vi "Read CategoriesChanged Event.vi"(8 "error in (no error)":errorcluster, 11 "VIStore in":refnum<class "VIStore.lvclass">) -> (0 "error out":errorcluster, 2 "CatList Changed Event":refnum<user-event>, 3 "VIStore out":refnum<class "VIStore.lvclass">)   [LabVIEW 2015, in "VI App Store.lvlib" / "VIStore.lvclass"]
uses:
  VIStore.lvclass
  VIStore.lvclass/VIStore.ctl
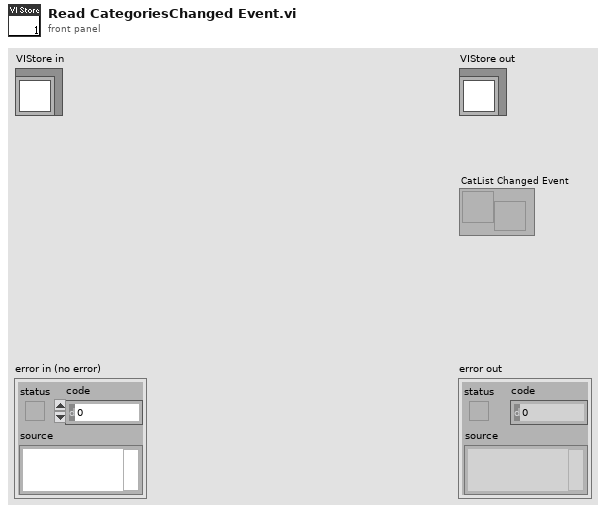
[diagram p1: front panel]
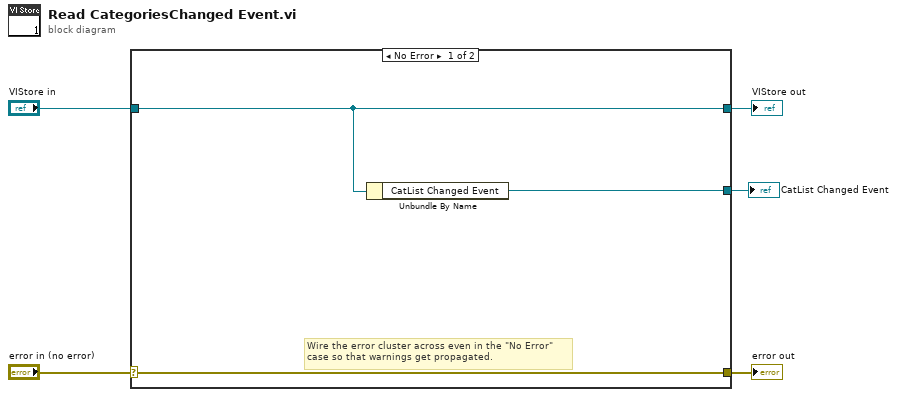
[diagram p0: block diagram]
diagram:
  n1 = case shown="No Error" "error in (no error)" {
    selector: "error in (no error)" -> [w8 w10]
    tunnel: [w8 w10] -> w4
    tunnel: [w7 w9] -> w2
    tunnel: "VIStore in" -> [w7 w9]
    tunnel: [w6 _] -> w1
    frame No Error {
      # "Wire the error cluster across even in the \"No Error\"\ncase so that warnings get propagated."
      n2 = Unbundle By Name(w7) -> ("CatList Changed Event"=w6:refnum<user-event>)
    }
    frame Error {
    }
  }
  "error out" <- w4
  "VIStore out" <- w2
  "CatList Changed Event" <- w1
